vi "ChannelDefine.vi"(9 "Search Term":string="cDAQ", 10 "Indices":i32[](array[numeric]), 11 "Tasks":tag[](array[tag])) -> (1 "Names":string[](array[string]), 2 "Tasks&Ind":T1[](array[typedef]), 3 "Remaining":T1[](array[typedef]))   [LabVIEW 2013]
uses:
  Channels_and_Index.ctl
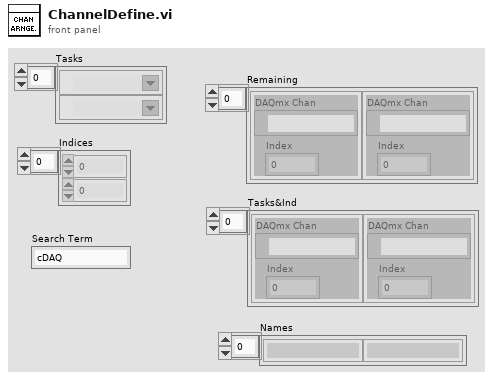
[diagram p1: front panel]
types:
  T1 = typedef "Channels_and_Index.ctl" = cluster{"DAQmx Chan":tag, "Index":i32}
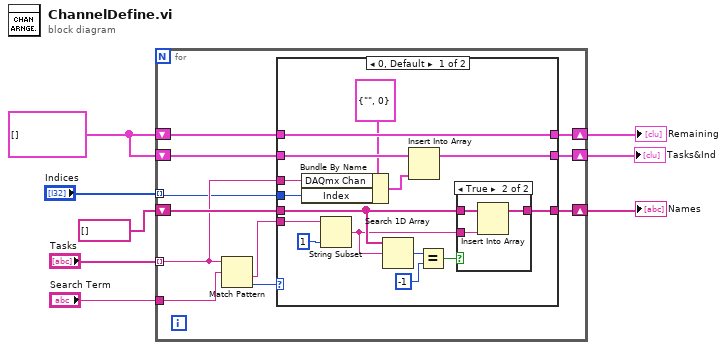
[diagram p0: block diagram]
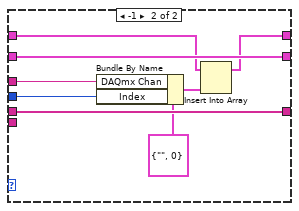
[diagram p3: hidden frame]
diagram:
  w3 = T1[] [] ("Array 6")
  n1 = for {
    shift-right: [w16] -> w4
    shift-left: w3 -> [w18]
    shift-right: [w15] -> w6
    shift-left: w3 -> [w17]
    shift-right: [w12] -> w5
    shift-left: string[] [] ("Array 7") -> [w14]
    tunnel: "Indices" -> [w10] mode=indexing
    tunnel: "Tasks" -> [w11] mode=indexing
    tunnel: "Search Term" -> [w9]
    n2 = Match Pattern(string=w11, regular expression=w9) -> (after substring=w13:string, offset past match=w19:i32)  [unwired: 1 in, 2 out]
    n3 = case shown="0, Default" w19 {
      tunnel: w11 -> [w21 w40]
      tunnel: w18 -> [w34 w45]
      tunnel: w17 -> [w33 w46]
      tunnel: [w34 w44] -> w16
      tunnel: [w32 w46] -> w15
      tunnel: w14 -> [w28 w43]
      tunnel: w13 -> [w30 _]
      tunnel: [w29 w43] -> w12
      tunnel: w10 -> [w20 w39]
      frame 0, Default {
        n4 = Bundle By Name(cluster=T1 {"DAQmx Chan"="", "Index"=0} ("Indexes"), "DAQmx Chan"=w21, "Index"=w20) -> (w22:T1)
        n5 = String Subset(string=w30, length (rest)=1 ("length (rest)")) -> (substring=w27:string)  [unwired: 1 in]
        n6 = Search 1D Array(1D array=w28, element=w27) -> (index of element=w26:i32)  [unwired: 1 in]
        n7 = Insert Into Array(array=w33, new element=w22) -> (w32:T1[])  [unwired: 1 in]
        n8 = Equal?(x=w26, y=-1) -> (x = y?=w24:bool)
        n9 = case shown="True" w24 {
          tunnel: [w35 w38] -> w29
          tunnel: w28 -> [w35 w37]
          tunnel: w27 -> [_ w36]
          frame False {
          }
          frame True {
            n10 = Insert Into Array(array=w37, new element=w36) -> (w38:string[])  [unwired: 1 in]
          }
        }
      }
      frame -1 {
        n11 = Bundle By Name(cluster=T1 {"DAQmx Chan"="", "Index"=0} ("Indexes"), "DAQmx Chan"=w40, "Index"=w39) -> (w41:T1)
        n12 = Insert Into Array(array=w45, new element=w41) -> (w44:T1[])  [unwired: 1 in]
      }
    }
  }
  "Tasks&Ind" <- w6
  "Names" <- w5
  "Remaining" <- w4
